vi "Reset.vi"(8 "error in (no error)":errorcluster, 11 "VISA resource name":refnum<visa-resource-name>) -> (0 "error out":errorcluster, 3 "VISA resource name out":refnum<visa-resource-name>)   [LabVIEW 2020, in "Library Instrument & Equipement.lvlib" / "Library Multimeter.lvlib" / "RIGOL DM3058.lvlib"]
doc: "Resets the instrument and then sends a set of default setup commands to the instrument."
uses:
  RIGOL DM3058.lvlib
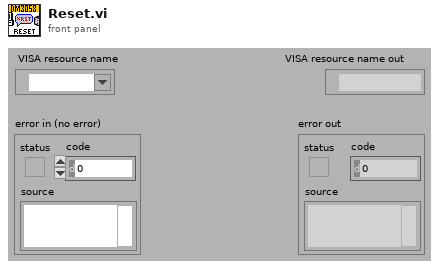
[diagram p1: front panel]
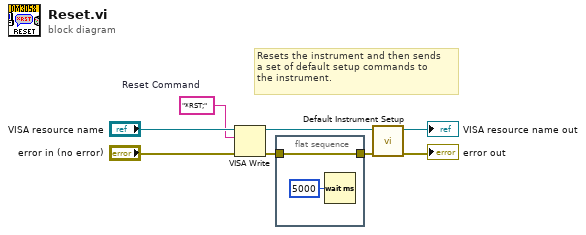
[diagram p0: block diagram]
diagram:
  w6 = "*RST;"  # Reset Command
  # "Resets the instrument and then sends \na set of default setup commands to \nthe instrument."
  n1 = VISA Write(VISA resource name="VISA resource name", write buffer=w6, error in (no error)="error in (no error)") -> (VISA resource name out=w5:refnum<visa-resource-name>, error out=w2:errorcluster)  [unwired: 1 out]
  n2 = flat-sequence {
    tunnel: w2 -> [w10]
    tunnel: [w10] -> w1
    frame #0 {
      n3 = Wait (ms)(milliseconds to wait=u32 5000) -> ()  [unwired: 1 out]
    }
  }
  n4 = call "Default Instrument Setup.vi"("error in (no error)"=w1, "VISA resource name"=w5) -> ("error out"=→"error out":errorcluster, "VISA resource name out"=→"VISA resource name out":refnum<visa-resource-name>)  [unwired: 8 out]
